vi "Variables_Locales.vi"() -> ()   [LabVIEW 2020]
panel:
  in  "Boolean":bool
  out "Waveform Chart 2":dbl(graph)
  out "Waveform Chart":dbl(graph)
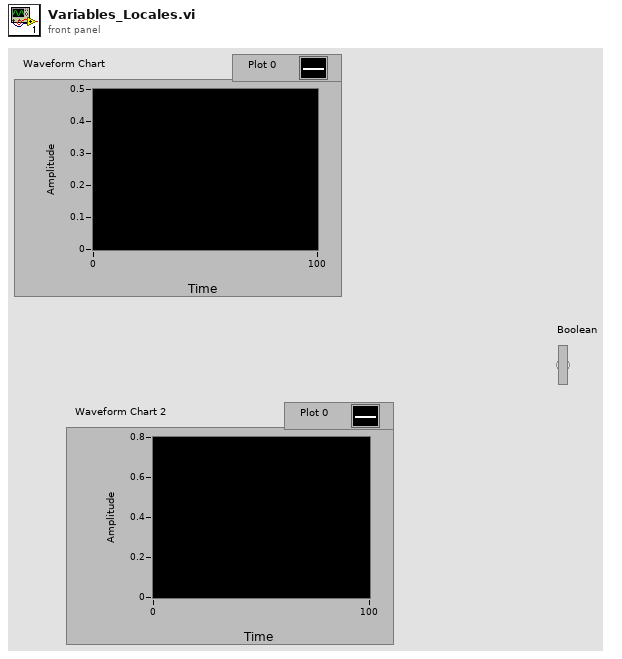
[diagram p1: front panel]
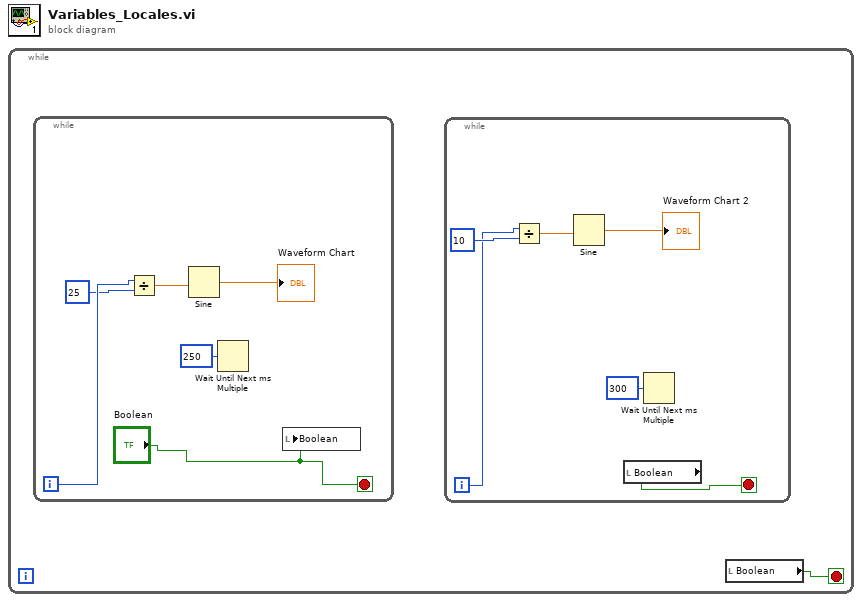
[diagram p0: block diagram]
diagram:
  n1 = while {
    stop <- w1 stop-if-true
    n2 = while {
      i -> [w11]
      stop <- "Boolean" stop-if-true
      n3 = Divide(x=w11, y=25) -> (x/y=w12:dbl)
      n4 = Sine(x=w12) -> (sin(x)=→"Waveform Chart":dbl)
      n5 = Wait Until Next ms Multiple(millisecond multiple=u32 250) -> ()  [unwired: 1 out]
      n6 = local write "Boolean"("Boolean") -> ()
    }
    n7 = while {
      i -> [w3]
      stop <- w2 stop-if-true
      n8 = Divide(x=w3, y=10) -> (x/y=w6:dbl)
      n9 = Sine(x=w6) -> (sin(x)=→"Waveform Chart 2":dbl)
      n10 = local read "Boolean"() -> (w2:bool)
      n11 = Wait Until Next ms Multiple(millisecond multiple=u32 300) -> ()  [unwired: 1 out]
    }
    n12 = local read "Boolean"() -> (w1:bool)
  }
